vi "Discovery FGV.vi"(0 "action":enum16{"Initialize", "Get"}(ring)=enum."Get", 7 "data in":T1) -> (8 "data out":T1)   [LabVIEW 2020, in "epl-network.lvlib"]
uses:
  epl-network.lvlib
  Discovery FGV.ctl
  Discovered Host.ctl
  Public/Discovery/Typedefs/Server Beacon.ctl
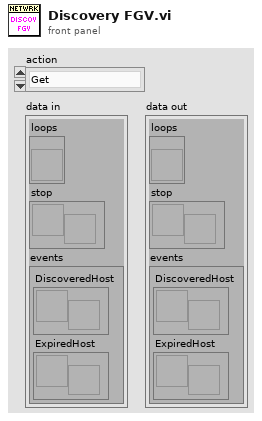
[diagram p1: front panel]
types:
  T1 = typedef "epl-network.lvlib/Discovery FGV.ctl" = cluster{"loops":refnum<vi>, "stop":refnum<notifier>, "events":cluster{"DiscoveredHost":refnum<user-event>, "ExpiredHost":refnum<user-event>}}
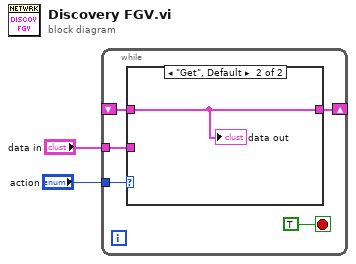
[diagram p0: block diagram]
diagram:
  n1 = while {
    shift-right: [w4] -> _
    shift-left: _ -> [w6]
    tunnel: "action" -> [w5]
    tunnel: "data in" -> [w3]
    stop <- TRUE stop-if-true
    n2 = case shown="\"Get\", Default" w5 {
      tunnel: w6 -> [_ w9]
      tunnel: [w8 w9] -> w4
      tunnel: w3 -> [w8 _]
      frame "Initialize" {
      }
      frame "Get", Default {
        "data out" <- w9
      }
    }
  }
